vi "Create HH Scope Page.vi"(8 "error in (no error)":errorcluster, 11 "Section Ptr":T1 format="%.0x") -> (0 "error out":errorcluster, 3 "Parent Ref out":T1 format="%.0x")   [LabVIEW 2016, in "DCM System Explorer.lvlib"]
uses:
  DCM System Explorer.lvlib
  <vilib>/NI Veristand/Custom Device API/Custom Device Item Ref.ctl
  <vilib>/NI Veristand/Custom Device API/Custom Device Channel Type.ctl
  <vilib>/NI Veristand/Custom Device API/Custom Device Waveform.ctl
  <vilib>/NI Veristand/Custom Device API/Custom Device Waveform DataType.ctl
  Shared/DCM Constants and GUIDs.vi
  DCM Shared.lvlib
  <vilib>/NI VeriStand/Custom Device API/Custom Device API.lvlib
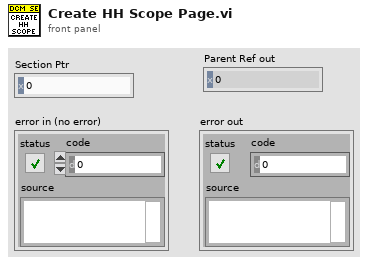
[diagram p1: front panel]
types:
  T1 = typedef "Custom Device API.lvlib/Custom Device Item Ref.ctl" = u64
  T2 = typedef "Custom Device API.lvlib/Custom Device Channel Type.ctl" = enum16{"Input", "Output"}
  T3 = typedef "DCM Shared.lvlib/Channel.ctl" = cluster{"Name":string, "Units":string, "Default":dbl, "Description":string}
  T4 = typedef "Custom Device API.lvlib/Custom Device Waveform DataType.ctl" = enum16{"Double", "Complex Double"}
  T5 = typedef "Custom Device API.lvlib/Custom Device Waveform.ctl" = cluster{"Data Type":T4, "Units":string}
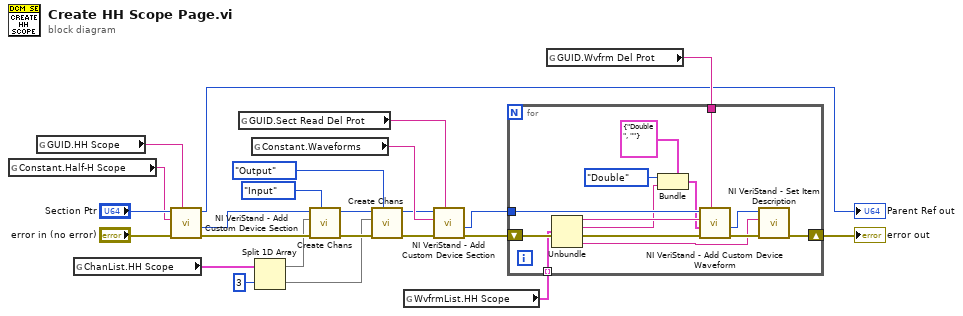
[diagram p0: block diagram]
diagram:
  n1 = global read "DCM Constants and GUIDs.vi" "Constant.Half-H Scope"() -> (w15:string)
  n2 = global read "DCM Constants and GUIDs.vi" "GUID.HH Scope"() -> (w14:string)
  n3 = global read "DCM Constants and GUIDs.vi" "ChanList.HH Scope"() -> (w5:T3[])
  n4 = call <vilib>:"NI VeriStand - Add Custom Device Section.vi"("GUID (Default Section)"=w14, "error in (no error)"="error in (no error)", "Section Name"=w15, "Parent Ref in"="Section Ptr") -> ("error out"=w12:errorcluster, "Section Ptr"=w11:T1, "Parent Ref out"=→"Parent Ref out":T1)  [unwired: 4 in, 1 out]
  n5 = global read "DCM Constants and GUIDs.vi" "GUID.Sect Read Del Prot"() -> (w19:string)
  n6 = global read "DCM Constants and GUIDs.vi" "Constant.Waveforms"() -> (w20:string)
  n7 = Split 1D Array(array=w5, index=3) -> (first subarray=w4:T3[], second subarray=w3:T3[])
  n8 = call "Create Chans.vi"("Type"=Custom_Device_Channel_Type."Input", "error in (no error)"=w12, "Channels"=w4, "Section Ptr"=w11) -> ("error out"=w7:errorcluster, "Section Ptr dup"=w9:T1)  [unwired: 4 in, 2 out]
  n9 = call "Create Chans.vi"("Type"=Custom_Device_Channel_Type."Output", "error in (no error)"=w7, "Channels"=w3, "Section Ptr"=w9) -> ("error out"=w6:errorcluster, "Section Ptr dup"=w8:T1)  [unwired: 4 in, 2 out]
  n10 = global read "DCM Constants and GUIDs.vi" "WvfrmList.HH Scope"() -> (w22:T3[])
  n11 = call <vilib>:"NI VeriStand - Add Custom Device Section.vi"("GUID (Default Section)"=w19, "error in (no error)"=w6, "Section Name"=w20, "Parent Ref in"=w8) -> ("error out"=w21:errorcluster, "Section Ptr"=w18:T1)  [unwired: 4 in, 2 out]
  n12 = global read "DCM Constants and GUIDs.vi" "GUID.Wvfrm Del Prot"() -> (w23:string)
  n13 = for {
    tunnel: w18 -> [w37]
    tunnel: w23 -> [w35]
    shift-right: [w32] -> w24
    shift-left: w21 -> [w36]
    tunnel: w22 -> [w29] mode=indexing
    n14 = Unbundle(w29) -> ("Name"=w28:string, "Units"=w26:string, "Description"=w25:string)  [unwired: 1 out]
    n15 = Bundle(cluster=T5 {"Data Type"=enum."Double", "Units"=""} ("Waveform"), "Data Type"=Custom_Device_Waveform_DataType."Double", "Units"=w26) -> (w27:T5)
    n16 = call <vilib>:"NI VeriStand - Add Custom Device Waveform.vi"("GUID (Default Waveform)"=w35, "error in (no error)"=w36, "Waveform"=w27, "Waveform Name"=w28, "Parent Ref in"=w37) -> ("error out"=w34:errorcluster, "Waveform Ref"=w33:T1)  [unwired: 3 in, 2 out]
    n17 = call <vilib>:"NI VeriStand - Set Item Description.vi"("error in (no error)"=w34, "Description"=w25, "Item Ref in"=w33) -> ("error out"=w32:errorcluster)  [unwired: 6 in, 2 out]
  }
  "error out" <- w24
